vi "ESC controller oneshot.vi"(3 "Error In":errorcluster, 4 "Output %":sgl min=0 max=100) -> (0 "Error out":errorcluster)   [LabVIEW 2021]
panel:
  out "Serial Port Name (Output)":string
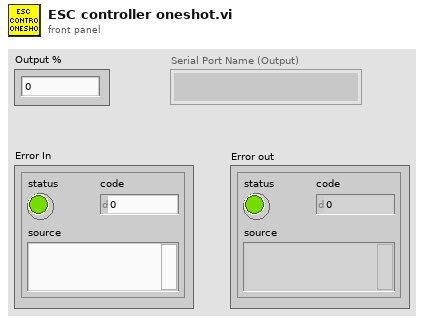
[diagram p1: front panel]
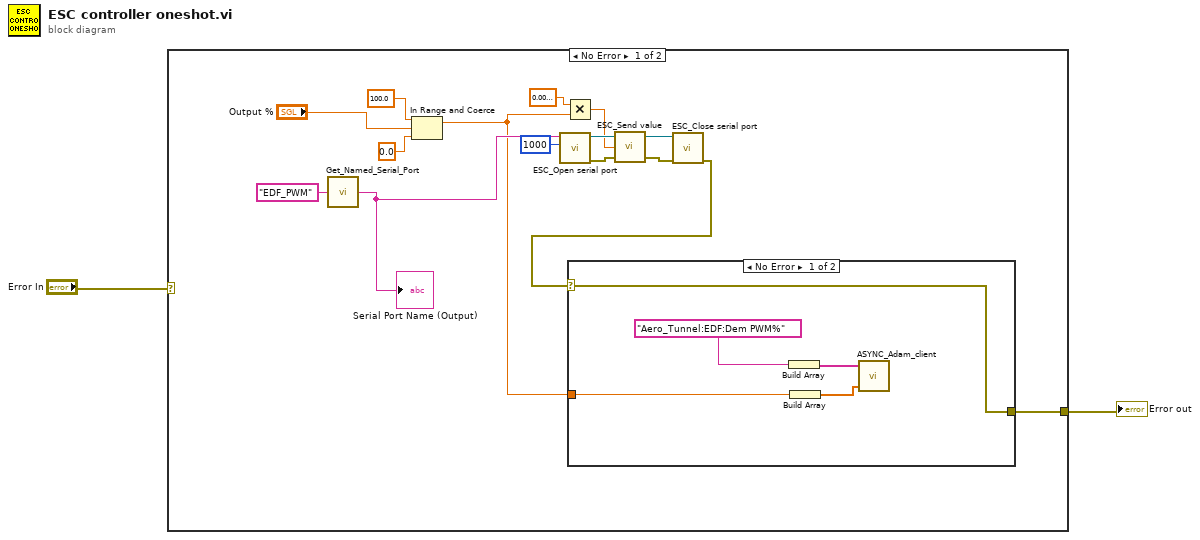
[diagram p0: block diagram]
diagram:
  n1 = case shown="No Error" "Error In" {
    selector: "Error In" -> [_ w24]
    tunnel: [w7 w24] -> w2
    frame No Error {
      n2 = call "Get_Named_Serial_Port.vi"("Serial Port Alias"="EDF_PWM") -> ("Serial Port Name"=w9:string)
      "Serial Port Name (Output)" <- w9
      n3 = In Range and Coerce(upper limit=100.0, x="Output %", lower limit=0.0) -> (coerced(x)=w3:dbl)  [unwired: 1 out]
      n4 = call "ESC_Open serial port.vi"("timeout (ms)"=u32 1000, "VISA resource name"=w9) -> ("Error out"=w16:errorcluster, "VISA resource name out"=w15:refnum<visa-resource-name>)  [unwired: 8 in]
      n5 = Multiply(x=sgl 0.01, y=w3) -> (x*y=w14:dbl)
      n6 = call "ESC_Send value.vi"("Error In"=w16, "Output (0...1)"=w14, "Port"=w15) -> ("Error Out"=w12:errorcluster, "Port out"=w11:refnum<visa-resource-name>)  [unwired: 1 out]
      n7 = call "ESC_Close serial port.vi"("Error in"=w12, "VISA resource name"=w11) -> ("Error out"=w10:errorcluster)  [unwired: 9 in]
      n8 = case shown="No Error" w10 {
        selector: w10 -> [w20 w23]
        tunnel: [w20 w23] -> w7
        tunnel: w3 -> [w18 _]
        frame No Error {
          n9 = Build Array("Aero_Tunnel:EDF:Dem PWM%") -> (w22:string[])
          n10 = Build Array(w18) -> (w19:dbl[])
          n11 = call "ASYNC_Adam_client.vi"("Values"=w19, "Channel Names"=w22) -> ()  [unwired: 1 in, 2 out]
        }
        frame Error {
        }
      }
    }
    frame Error {
    }
  }
  "Error out" <- w2
